vi "Freq-Mod_Prototype.vi"() -> ()   [LabVIEW 2012]
uses:
  <vilib>/rvi/eio/common/nirviEmuTemplateMethod_errors.vi
  <vilib>/eio/EIONode/EIONode.xnode
panel:
  in  "Sampling Frequency":i32=200000
  out "R (Amplitude)":fxp<+,7,1>
  out "Degrees":fxp<+,4,1>
  out "F Graph":fxp<+,14,17>
  in  "Time Constant":fxp<+,10,7>
  out "sin(z) [I16.2] 2":fxp<+/-,10,1>
  in  "alpha [U16.-2] 2":fxp<+,8,2>=0.046875
  in  "phase setpoint 2":fxp<+/-,6,2>=1.5 format="%#_3g"
  in  "dec1":i16=1
  in  "dec2":i16
  in  "stages":i8=1
  in  "decimation":i16=1024
  in  "K Constant":fxp<+,8,0>=0.0234375
  in  "Nominal Freq\nLIA":fxp<+,8,0>=0.203125
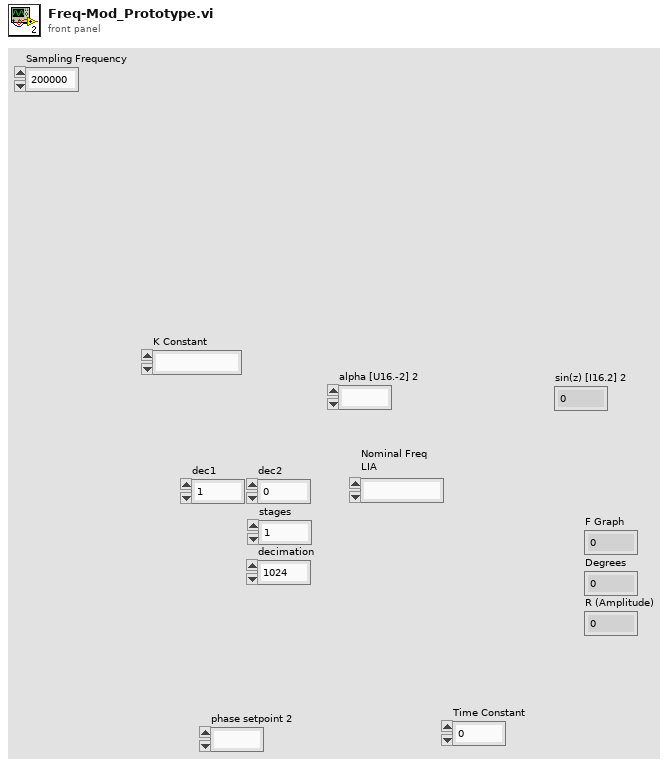
[diagram p1: front panel]
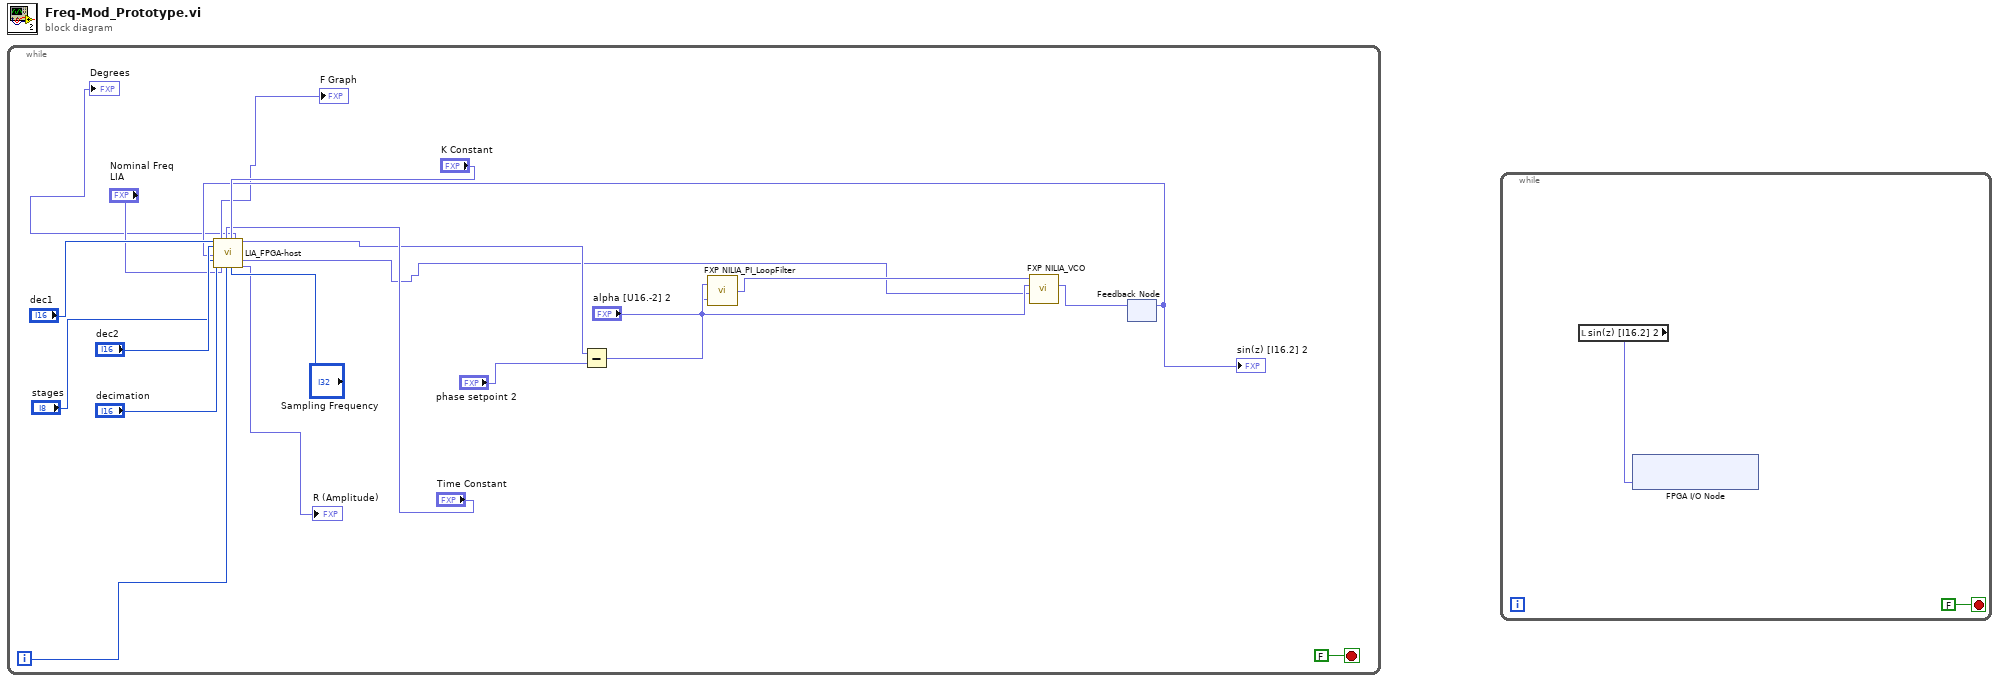
[diagram p0: block diagram]
diagram:
  n1 = while {
    i -> [w4]
    stop <- FALSE stop-if-true
    n2 = feedback #1() -> (w5:fxp<+/-,16,2>)  [unwired: 1 in]
    "sin(z) [I16.2] 2" <- w5
    n3 = call "LIA_FPGA-host.vi"("dec1"="dec1", "dec2"="dec2", "Ref Signal"=w5, "stages"="stages", "decimation"="decimation", "nominal freq  (LIA)"="Nominal Freq\nLIA", "Filter Constant"="Time Constant", "While Loop Counter"=w4, "K"="K Constant", "Sampling Frequency"="Sampling Frequency") -> ("F graph"=→"F Graph":fxp<+,64,64>, "Degree"=→"Degrees":fxp<+,1,1>, "phase (pi)"=w11:fxp<+/-,16,2>, "Nominal Freq"=w7:fxp<+/-,64,32>, "R"=→"R (Amplitude)":fxp<+,1,1>)  [unwired: 1 in, 4 out]
    n4 = Subtract(x=w11, y="phase setpoint 2") -> (x-y=w12:fxp<+/-,17,3>)
    n5 = call "FXP NILIA_PI_LoopFilter.vi"("alpha [U16.-2]"="alpha [U16.-2] 2", "x [I16.2]"=w12) -> ("x+y [I32.17]"=w9:fxp<+/-,32,17>)  [unwired: 1 in]
    n6 = call "FXP NILIA_VCO.vi"("nominal freq [U16.0]"=w7, "Kv [U16.0]"="alpha [U16.-2] 2", "v [I32.17]"=w9) -> ("sin(z) [I16.2]"=w6:fxp<+/-,16,2>)  [unwired: 5 in, 3 out]
    n7 = feedback-in #1(w6) -> ()
  }
  n8 = while {
    stop <- FALSE stop-if-true
    n9 = local read "sin(z) [I16.2] 2"() -> (w23:fxp<+/-,10,1>)
    n10 = xnode "FPGA I/O Node"("Connector0/AO5"=w23) -> ()  [unwired: 1 in, 1 out]
  }
